vi "setTriggerSource_MVF.vi"(6 "TriggerSourceStrings":T1, 7 "TrigerModeName":string="CameraAttributes::Trigger::TriggerMode", 8 "error in":errorcluster, 9 "cam connected":bool, 10 "Settings.Trigger":T3, 11 "Session":T2) -> (0 "error out":errorcluster, 2 "Settings.Trigger  out":T3)   [LabVIEW 2020]
uses:
  shared/OnOffTypeDef.ctl
  <vilib>/userdefined/High Color/IMAQdx.ctl
  TriggerSource_TypDEF.ctl
  <resource>/objmgr/imaqdx.rc
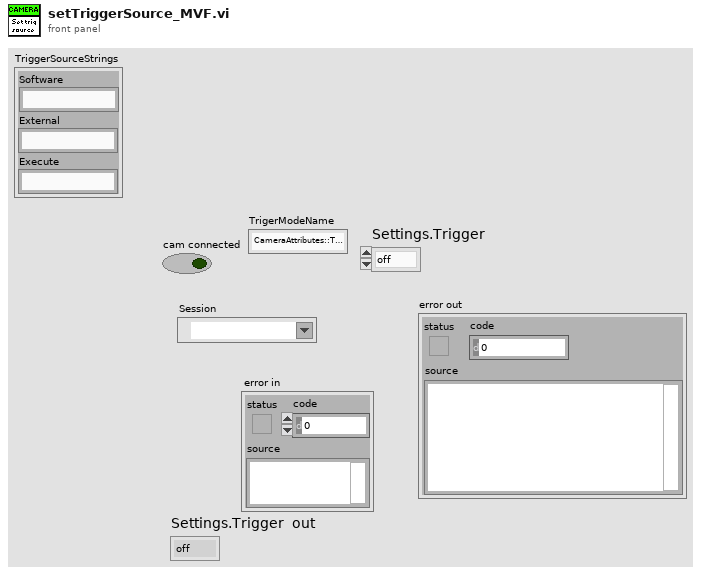
[diagram p1: front panel]
types:
  T1 = typedef "TriggerSource_TypDEF.ctl" = cluster{"Software":string, "External":string, "Execute":string}
  T2 = typedef "IMAQdx.ctl" = refnum<k21>
  T3 = typedef "OnOffTypeDef.ctl" = enum16{"off", "on"}
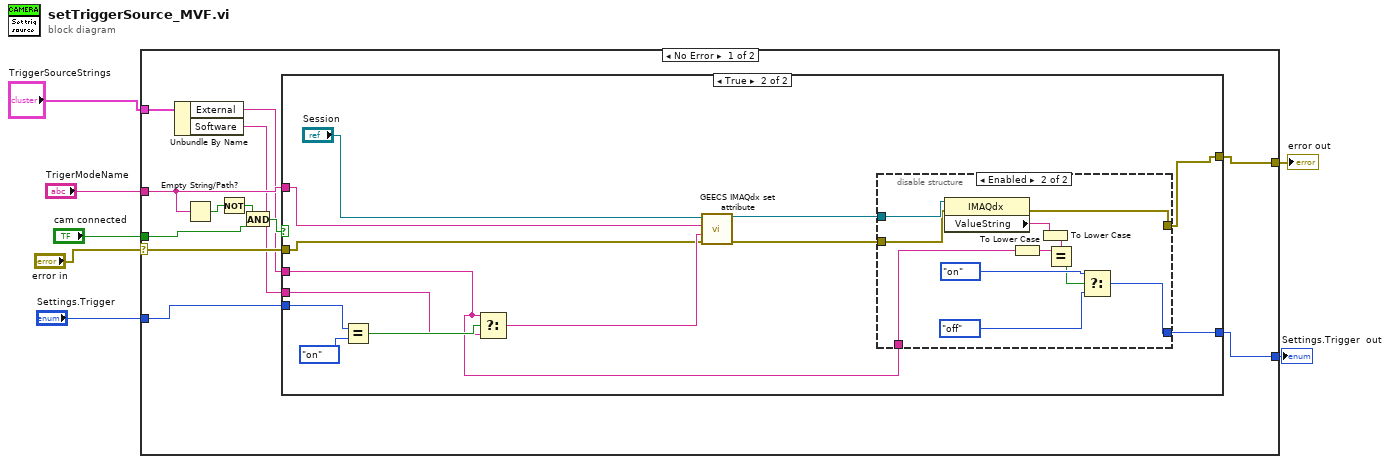
[diagram p0: block diagram]
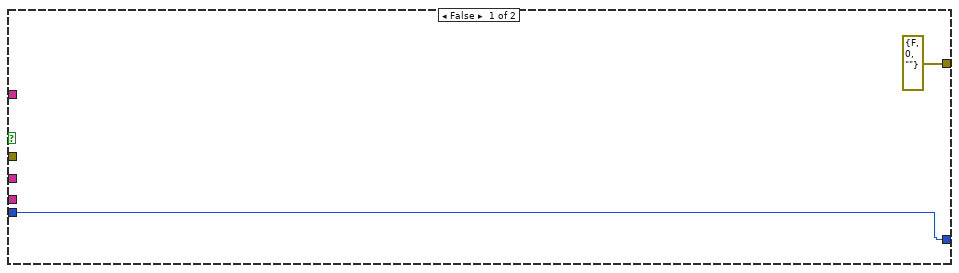
[diagram p2: hidden frame]
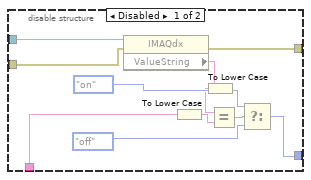
[diagram p3: hidden frame]
diagram:
  n1 = case shown="No Error" "error in" {
    selector: "error in" -> [w16 w57]
    tunnel: "cam connected" -> [w14 _]
    tunnel: "Settings.Trigger" -> [w19 _]
    tunnel: [w18 _] -> w5
    tunnel: "TrigerModeName" -> [w15 _]
    tunnel: [w17 w57] -> w3
    tunnel: "TriggerSourceStrings" -> [w10 _]
    frame No Error {
      n2 = Unbundle By Name(w10) -> ("External"=w8:string, "Software"=w9:string)
      n3 = Empty String/Path?(string/path=w15) -> (empty?=w13:bool)
      n4 = Not(x=w13) -> (.not. x?=w12:bool)
      n5 = And(x=w12, y=w14) -> (x .and. y?=w11:bool)
      n6 = case shown="True" w11 {
        tunnel: [errorcluster {"status"=FALSE, "code"=0, "source"=""} ("error out") w32] -> w17
        tunnel: [w20 w33] -> w18
        tunnel: w19 -> [w20 w31]
        tunnel: w15 -> [_ w25]
        tunnel: w9 -> [_ w22]
        tunnel: w8 -> [_ w23]
        tunnel: w16 -> [_ w24]
        frame False {
        }
        frame True {
          n7 = Equal?(x=w31, y=OnOffTypeDef."on" ("Settings.Trigger")) -> (x = y?=w34:bool)
          n8 = Select(t=w23, s=w34, f=w22) -> (s? t:f=w29:string)
          n9 = call "GEECS IMAQdx set attribute.vi"("error in (no error)"=w24, "Attribute value"=w29, "Attribute name"=w25, "Refnum in"="Session") -> ("error out"=w27:errorcluster, "Refnum out"=w28:T2)  [unwired: 6 in]
          n10 = disable-structure shown="Enabled" {
            disable-tunnel: [w45 w48] -> w33
            disable-tunnel: [w44 w54] -> w32
            disable-tunnel: w28 -> [w39 w56]
            disable-tunnel: w27 -> [w38 w55]
            disable-tunnel: w23 -> [w35 w47]
            frame Disabled {
              n11 = property class="IMAQdx"(reference=w39, error in=w38) -> (error out=w44:errorcluster, "ValueString"=w43:string)  [unwired: 1 out]
              n12 = To Lower Case(string=w35) -> (all lower case string=w36:string)
              n13 = To Lower Case(string=w43) -> (all lower case string=w37:string)
              n14 = Equal?(x=w37, y=w36) -> (x = y?=w42:bool)
              n15 = Select(t=OnOffTypeDef."on" ("Settings.Trigger"), s=w42, f=OnOffTypeDef."off" ("Settings.Trigger")) -> (s? t:f=w45:T3)
            }
            frame Enabled {
              n16 = property class="IMAQdx"(reference=w56, error in=w55) -> (error out=w54:errorcluster, "ValueString"=w53:string)  [unwired: 1 out]
              n17 = To Lower Case(string=w47) -> (all lower case string=w46:string)
              n18 = To Lower Case(string=w53) -> (all lower case string=w52:string)
              n19 = Equal?(x=w52, y=w46) -> (x = y?=w49:bool)
              n20 = Select(t=OnOffTypeDef."on" ("Settings.Trigger"), s=w49, f=OnOffTypeDef."off" ("Settings.Trigger")) -> (s? t:f=w48:T3)
            }
          }
        }
      }
    }
    frame Error {
    }
  }
  "Settings.Trigger  out" <- w5
  "error out" <- w3
